vi "Reverse Integer.vi"(8 "Error Input":errorcluster, 11 "Input":i32) -> (0 "Error Output":errorcluster, 3 "Output":i32)   [LabVIEW 2024]
doc: "This VI reverse the input integer."
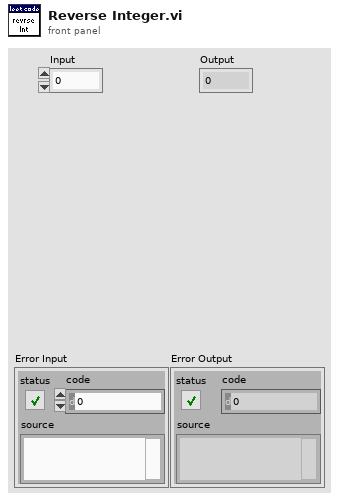
[diagram p1: front panel]
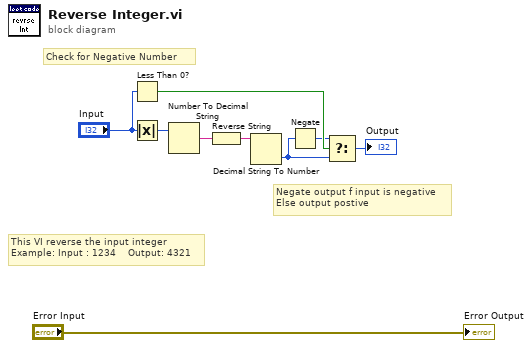
[diagram p0: block diagram]
diagram:
  # "This VI reverse the input integer\nExample: Input : 1234    Output: 4321"
  # "Negate output f input is negative\nElse output postive"
  # "Check for Negative Number"
  n1 = Less Than 0?(x="Input") -> (x < 0?=w9:bool)
  n2 = Absolute Value(x="Input") -> (abs(x)=w5:i32)
  n3 = Number To Decimal String(number=w5) -> (decimal integer string=w3:string)  [unwired: 1 in]
  n4 = Reverse String(1:w3) -> (0:w2:string)
  n5 = Decimal String To Number(string=w2) -> (number=w7:i32)  [unwired: 2 in, 1 out]
  n6 = Negate(x=w7) -> (-x=w8:i32)
  n7 = Select(t=w8, s=w9, f=w7) -> (s? t:f=→"Output":i32)
  "Error Output" <- "Error Input"
